vi "Discover Unique Names of Dependencies.vi"(0 "Export In":refnum<class "Export.lvclass">) -> (4 "Export Out":refnum<class "Export.lvclass">)   [LabVIEW 2017, in "CL_G3_VIComponentBuilder.lvlib" / "Export.lvclass"]
doc: "Interrogates this exports dependencies for thier unique names (as opposed to the product name of the dependency). The unique names are used when assembling the working set of exports in order to prevent name collisions and allow the build analyzer to determine the build order.\n<RequiredOverrideReason>Each export type by definition can have dependencies. The way in which an export finds what other exports it depends on is export type specific.</RequiredOverrideReason>\n<MustCallParent>The parent makes the text all lower case to ensure that lookup is successful</MustCallParent>"
uses:
  Export.lvclass
  Export.lvclass/Export.ctl
  Accessors/Read Dependencies' Unique Names.vi
  Accessors/Read Export Operation Errors.vi
  Accessors/Write Dependencies' Unique Names.vi
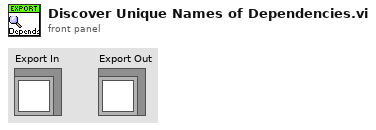
[diagram p1: front panel]
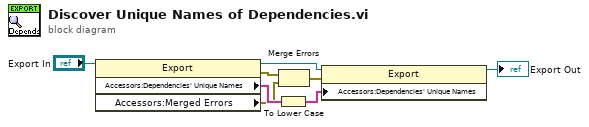
[diagram p0: block diagram]
diagram:
  n1 = property class="Export"(reference="Export In") -> (reference out=w7:refnum<class "Export.lvclass">, error out=w3:errorcluster, "Accessors:Dependencies' Unique Names"=w5:string[], "Accessors:Merged Errors"=w1:errorcluster)  [unwired: 1 in]
  n2 = To Lower Case(string=w5) -> (all lower case string=w4:string[])
  n3 = Merge Errors(w3, w1) -> (w2:errorcluster)
  n4 = property class="Export"(reference=w7, error in=w2, "Accessors:Dependencies' Unique Names"=w4) -> (reference out=→"Export Out":refnum<class "Export.lvclass">)  [unwired: 1 out]
